vi "Password Condition (SubVI).vi"(1 "Y":bool, 2 "X":bool) -> (0 "Password Condition":string)   [LabVIEW 2015]
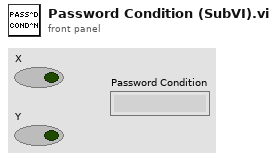
[diagram p1: front panel]
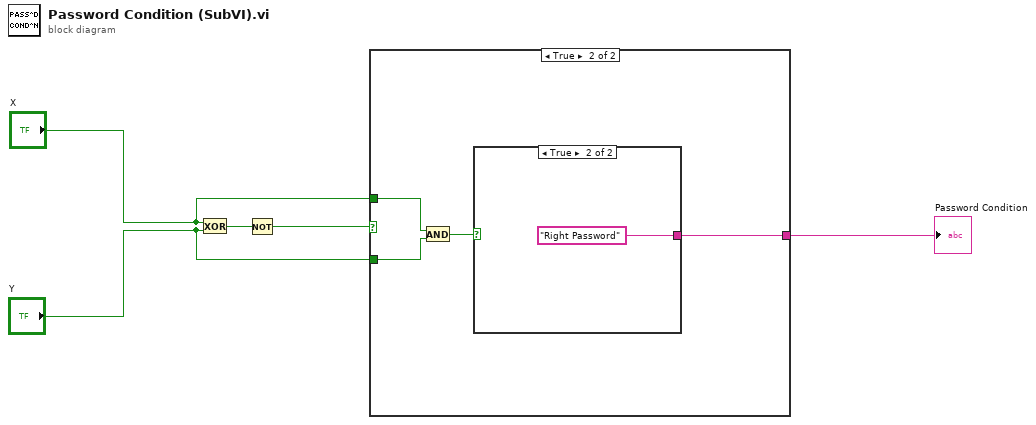
[diagram p0: block diagram]
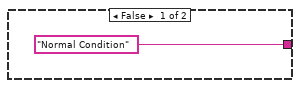
[diagram p2: hidden frame]
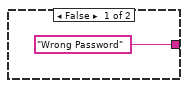
[diagram p3: hidden frame]
diagram:
  n1 = Exclusive Or(1:"Y", 2:"X") -> (0:w1:bool)
  n2 = Not(x=w1) -> (.not. x?=w2:bool)
  n3 = case shown="True" w2 {
    tunnel: ["Normal Condition" w10] -> w3
    tunnel: "X" -> [_ w8]
    tunnel: "Y" -> [_ w7]
    frame False {
    }
    frame True {
      n4 = And(x=w8, y=w7) -> (x .and. y?=w9:bool)
      n5 = case shown="True" w9 {
        tunnel: ["Wrong Password" "Right Password"] -> w10
        frame False {
        }
        frame True {
        }
      }
    }
  }
  "Password Condition" <- w3
